vi "MMI_Intelligent_StrDismantle.vi"(1 "LogEvent":refnum<vi>, 2 "VCI_CAN_OBJ_R":T1) -> (0 "MMI_ItelligentCmdCluster":T2 {"下一拥堵路段的长度" scale=0.0..100.0; "距离下一拥堵路段距离" scale=0.0..100.0; "下一路段拥堵等级" items=["正常", "等级1", "等级2", "等级3"]; "当前拥堵路段剩余长度" scale=0.0..100.0; "当前路段拥堵等级" items=["正常", "等级1", "等级2", "等级3"]; "当前行驶路况" items=["普通路况", "高速路况", "其它"]})   [LabVIEW 2013]
uses:
  Log.ctl
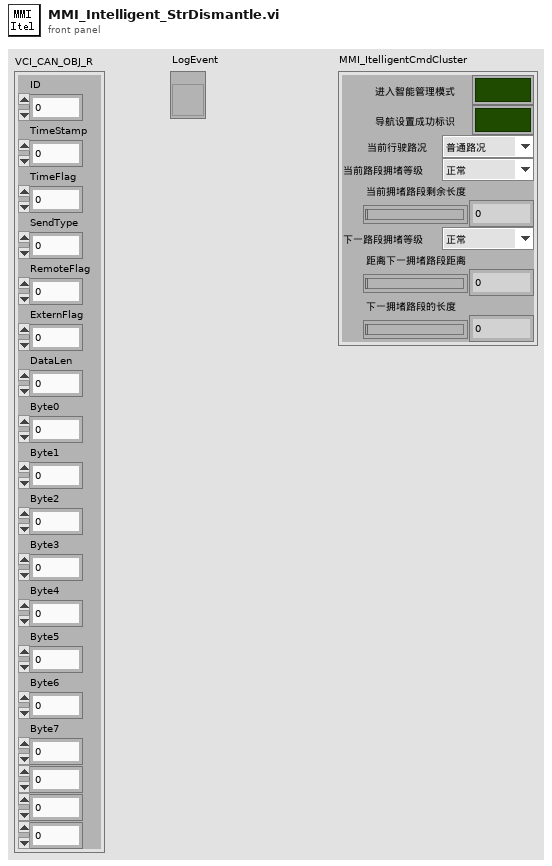
[diagram p1: front panel]
types:
  T1 = cluster{"ID":u32, "TimeStamp":u32, "TimeFlag":u8, "SendType":u8, "RemoteFlag":u8, "ExternFlag":u8, "DataLen":u8, "Byte0":u8, "Byte1":u8, "Byte2":u8, "Byte3":u8, "Byte4":u8, "Byte5":u8, "Byte6":u8, "Byte7":u8, u8, u8, u8}
  T2 = cluster{"进入智能管理模式":bool, "导航设置成功标识":bool, "当前行驶路况":u16, "当前路段拥堵等级":u16, "当前拥堵路段剩余长度":i32, "下一路段拥堵等级":u16, "距离下一拥堵路段距离":dbl, "下一拥堵路段的长度":dbl}
  T3 = typedef "Log.ctl" = cluster{"Event":string, "Value":variant}
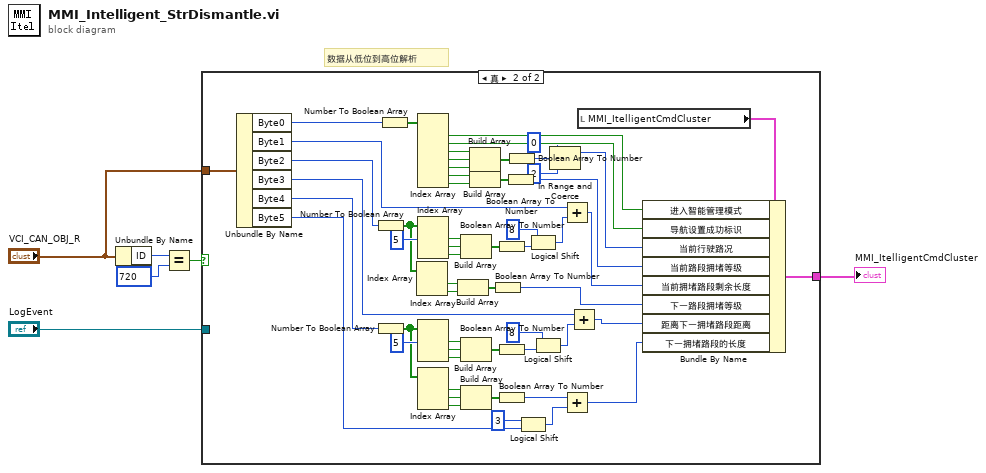
[diagram p0: block diagram]
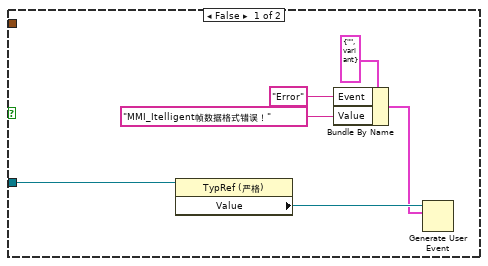
[diagram p2: hidden frame]
diagram:
  # "数据从低位到高位解析"
  n1 = Unbundle By Name("VCI_CAN_OBJ_R") -> ("ID"=w5:u32)
  n2 = Equal?(x=w5, y=u16 720) -> (x = y?=w3:bool)
  n3 = case shown="真" w3 {
    tunnel: [_ w67] -> w6
    tunnel: "VCI_CAN_OBJ_R" -> [_ w19]
    tunnel: "LogEvent" -> [w7 _]
    frame False {
      n4 = property class="TypRef (严格)"(reference=w7) -> ("Value"=w12:refnum<user-event>)  [unwired: 1 in, 2 out]
      n5 = Bundle By Name(cluster=T3 {"Event"="", "Value"=variant} ("Log"), "Event"="Error", "Value"="MMI_Itelligent帧数据格式错误！" ("消息")) -> (w9:T3)
      n6 = Generate User Event(user event=w12, event data cluster=w9) -> ()  [unwired: 2 in, 2 out]
    }
    frame True {
      n7 = Unbundle By Name(w19) -> ("Byte0"=w18:u8, "Byte1"=w17:u8, "Byte2"=w16:u8, "Byte3"=w15:u8, "Byte4"=w14:u8, "Byte5"=w13:u8)
      n8 = Number To Boolean Array(number=w16) -> (Boolean array=w42:bool[])
      n9 = Number To Boolean Array(number=w14) -> (Boolean array=w24:bool[])
      n10 = Number To Boolean Array(number=w18) -> (Boolean array=w66:bool[])
      n11 = Index Array(array=w42) -> (element #1=w40:bool, element #2=w41:bool)  [unwired: 2 in]
      n12 = Index Array(array=w66) -> (element #1=w65:bool, element #2=w64:bool, element #3=w63:bool, element #4=w62:bool, element #5=w59:bool, element #6=w55:bool, element #7=w54:bool)  [unwired: 7 in]
      n13 = Index Array(array=w42, index #1=5 ("索引")) -> (element #1=w49:bool, element #2=w50:bool, element #3=w48:bool)  [unwired: 2 in]
      n14 = Index Array(array=w24, index #1=5 ("索引")) -> (element #1=w34:bool, element #2=w33:bool, element #3=w31:bool)  [unwired: 2 in]
      n15 = Index Array(array=w24) -> (element #1=w26:bool, element #2=w27:bool, element #3=w28:bool)  [unwired: 3 in]
      n16 = Build Array(w40, w41) -> (w39:bool[])
      n17 = Build Array(w49, w50, w48) -> (w47:bool[])
      n18 = Build Array(w34, w33, w31) -> (w35:bool[])
      n19 = Build Array(w26, w27, w28) -> (w25:bool[])
      n20 = Build Array(w63, w62, w59) -> (w61:bool[])
      n21 = Build Array(w55, w54) -> (w53:bool[])
      n22 = Boolean Array To Number(Boolean array=w39) -> (number=w38:u32)
      n23 = Boolean Array To Number(Boolean array=w47) -> (number=w46:u32)
      n24 = Boolean Array To Number(Boolean array=w35) -> (number=w36:u32)
      n25 = Boolean Array To Number(Boolean array=w25) -> (number=w22:u32)
      n26 = Boolean Array To Number(Boolean array=w53) -> (number=w52:u32)
      n27 = Boolean Array To Number(Boolean array=w61) -> (number=w60:u32)
      n28 = Logical Shift(y=i16 3, x=w13) -> (x << y=w21:u8)
      n29 = Logical Shift(y=u8 8, x=w46) -> (x << y=w44:u32)
      n30 = Logical Shift(y=u8 8, x=w36) -> (x << y=w30:u32)
      n31 = In Range and Coerce(upper limit=u32 0 ("上限"), x=w60, lower limit=u32 2 ("下限")) -> (coerced(x)=w58:u32)  [unwired: 1 out]
      n32 = Add(x=w17, y=w44) -> (x+y=w43:u32)
      n33 = Add(x=w22, y=w21) -> (x+y=w20:u32)
      n34 = Add(x=w15, y=w30) -> (x+y=w29:u32)
      n35 = local read "MMI_ItelligentCmdCluster"() -> (w68:T2)
      n36 = Bundle By Name(cluster=w68, "进入智能管理模式"=w65, "导航设置成功标识"=w64, "当前行驶路况"=w58, "当前路段拥堵等级"=w52, "当前拥堵路段剩余长度"=w43, "下一路段拥堵等级"=w38, "距离下一拥堵路段距离"=w29, "下一拥堵路段的长度"=w20) -> (w67:T2)
    }
  }
  "MMI_ItelligentCmdCluster" <- w6
